vi "Add_sample_in_AO_DO_tasks_with_odd_number_of_samples.vi"(6 "Dummy Gate Waveform IN":waveform(i16), 7 "Black list (devices unable to output odd number of samples)":string[](array[string])=["PCI-6110"], 8 "error in (no error)":errorcluster, 9 "Gate Waveform (Digital) IN":digitalwaveform(waveform)={"t0"=timestamp(0 s since 1904-01-01), "dt"=0.0, "Y"={"transitions"=[], "data"=[]}, "error"={"status"=FALSE, "code"=37421928, "source"=""}}, 10 "Pockels Waveform IN":waveform(dbl), 11 "XY Waveform IN":waveform(dbl)[](array[waveform])) -> (0 "error out":errorcluster, 1 "Gate Waveform (Digital) OUT":digitalwaveform(waveform)={"t0"=timestamp(0 s since 1904-01-01), "dt"=0.0, "Y"={"transitions"=[], "data"=[]}, "error"={"status"=FALSE, "code"=37421928, "source"=""}}, 2 "Pockels Waveform OUT":waveform(dbl), 3 "XY Waveform OUT":waveform(dbl)[](array[waveform]), 4 "Dummy Gate Waveform OUT":waveform(i16), 5 "Sample added at the end of each task?":bool)   [LabVIEW 2012]
uses:
  GFG/GFGbooleanGet.vi
  GFG/GFGstringGet.vi
  <vilib>/Waveform/DWDTOps.llb/DWDT Digital Size.vi
  <vilib>/Waveform/WDTOps.llb/WDT Number of Waveform Samples DBL.vi
  <vilib>/Waveform/DWDTOps.llb/DWDT Digital to Boolean Array.vi
  <vilib>/Waveform/DTblOps.llb/DTbl Boolean Array to Digital.vi
  GFG/GFG library.lvlib
  <resource>/objmgr/daqmx.rc
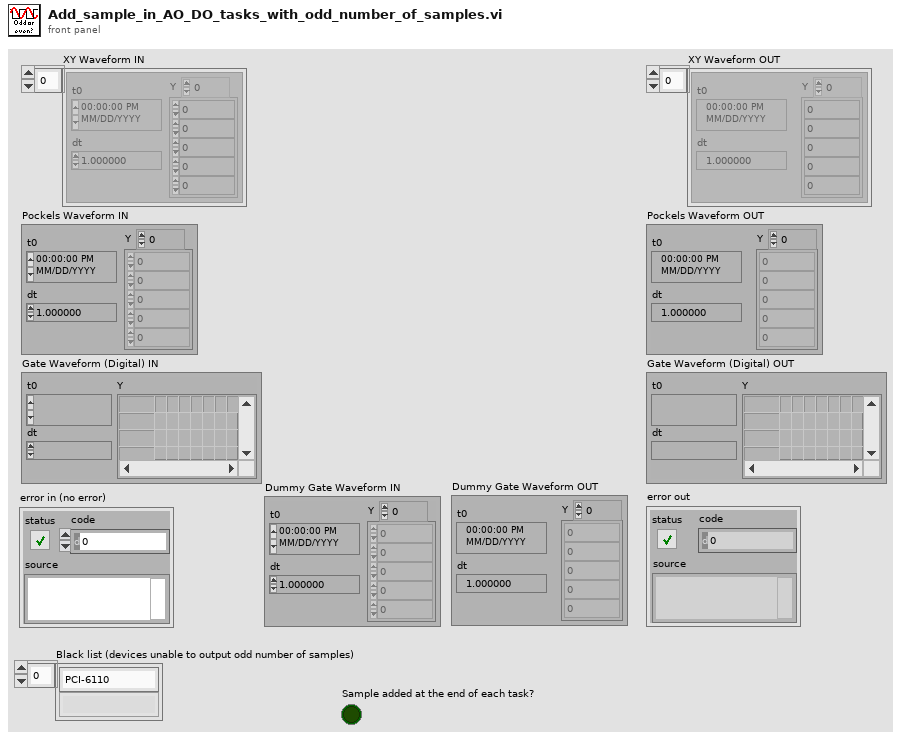
[diagram p1: front panel]
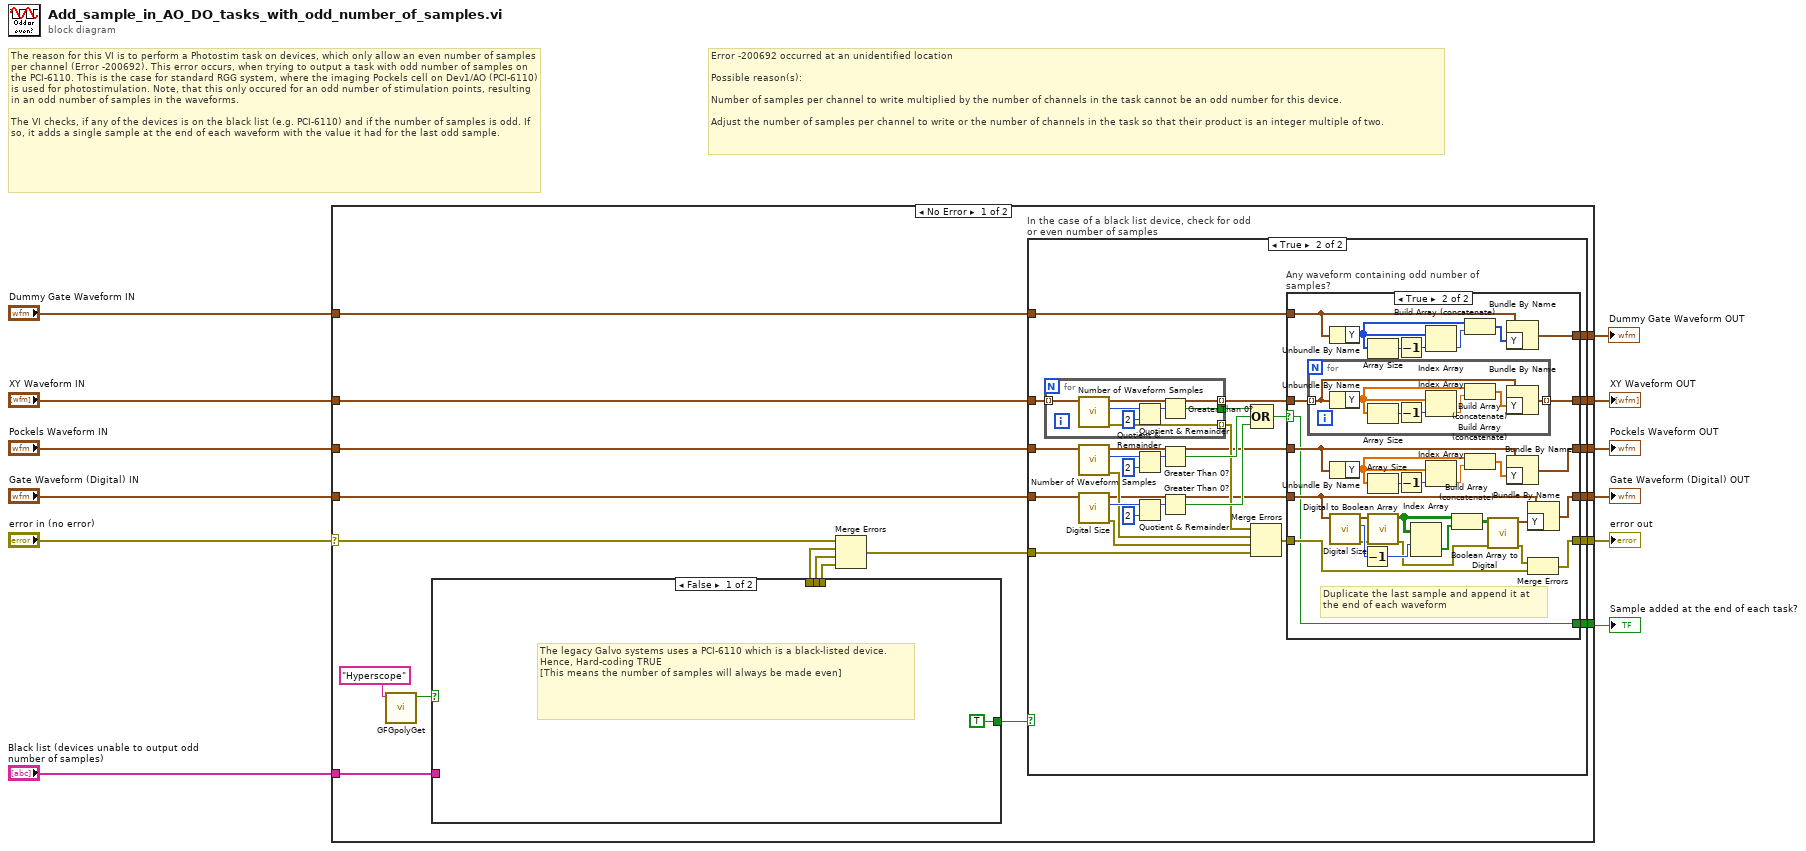
[diagram p0: block diagram]
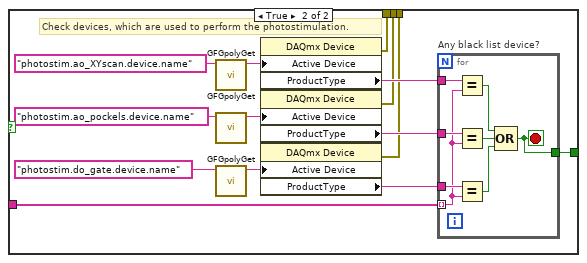
[diagram p2: hidden frame]
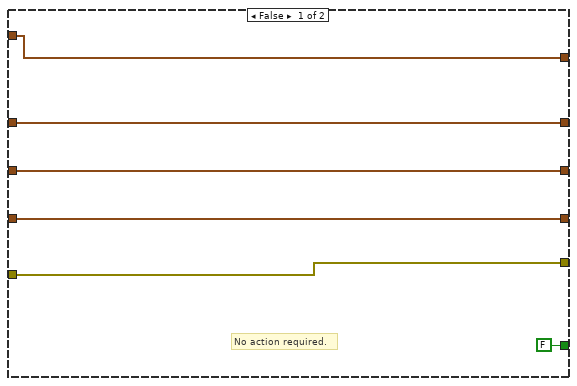
[diagram p3: hidden frame]
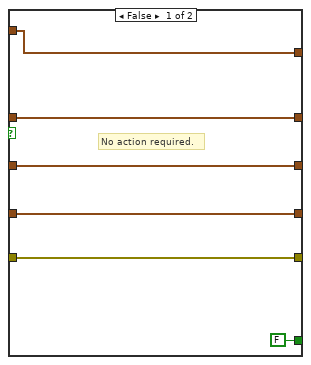
[diagram p4: hidden frame]
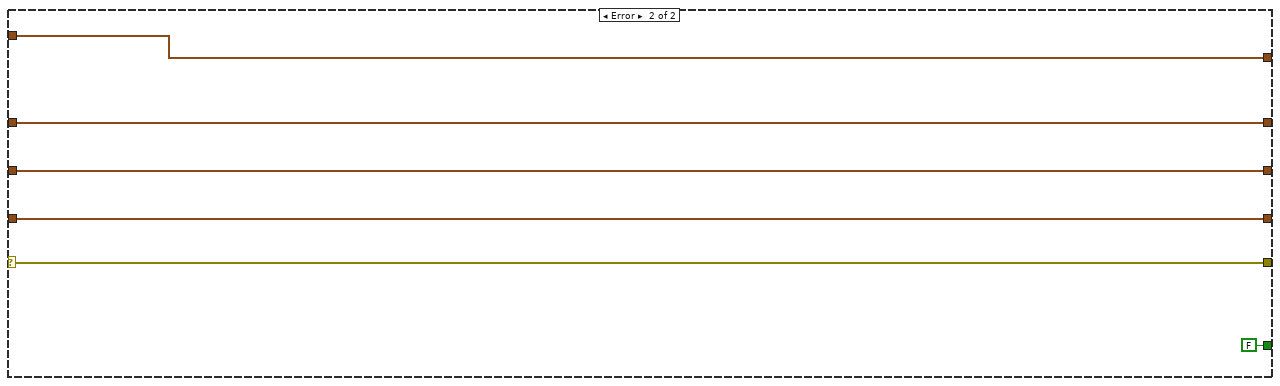
[diagram p5: hidden frame]
diagram:
  # "The reason for this VI is to perform a Photostim task on devices, which only allow an even number of samples per channel (Error -200692). This error occurs, when trying to output a task with odd number of samples on the PCI-6110. This is the case for standard RGG system, where the imaging Pockels cell on Dev1/AO (PCI-6110) is used for photostimulation. Note, that this only occured for an odd number of stimulation points, resulting in an odd number of samples in the waveforms.\n\nThe VI checks, if any of the devices is on the black list (e.g. PCI-6110) and if the number of samples is odd. If so, it adds a single sample at the end of each waveform with the value it had for the last odd sample."
  # "Error -200692 occurred at an unidentified location\n\nPossible reason(s):\n\nNumber of samples per channel to write multiplied by the number of channels in the task cannot be an odd number for this device. \n\nAdjust the number of samples per channel to write or the number of channels in the task so that their product is an integer multiple of two."
  n1 = case shown="No Error" "error in (no error)" {
    selector: "error in (no error)" -> [w27 w142]
    tunnel: "XY Waveform IN" -> [w26 w145]
    tunnel: "Pockels Waveform IN" -> [w25 w144]
    tunnel: "Gate Waveform (Digital) IN" -> [w24 w143]
    tunnel: [w22 w145] -> w11
    tunnel: [w21 w144] -> w10
    tunnel: [w20 w143] -> w9
    tunnel: [w19 w142] -> w8
    tunnel: "Black list (devices unable to output odd number of samples)" -> [w31 _]
    tunnel: [w17 FALSE] -> w3
    tunnel: "Dummy Gate Waveform IN" -> [w16 w140]
    tunnel: [w15 w140] -> w1
    frame No Error {
      n2 = call-poly "GFGpolyGet.vi"("Variable Name in"="Hyperscope") -> ("Boolean Value OUT"=w13:bool)  [unwired: 9 in, 1 out]
      n3 = case shown="False" w13 {
        tunnel: w31 -> [_ w40]
        tunnel: [_ w36] -> w30
        tunnel: [_ w35] -> w29
        tunnel: [_ w34] -> w28
        tunnel: [TRUE w33] -> w18
        frame False {
          # "The legacy Galvo systems uses a PCI-6110 which is a black-listed device. Hence, Hard-coding TRUE \n[This means the number of samples will always be made even]"
        }
        frame True {
          # "Check devices, which are used to perform the photostimulation."
          n4 = call-poly "GFGpolyGet.vi"("Variable Name in"="photostim.ao_XYscan.device.name") -> ("String"=w43:string)  [unwired: 9 in, 1 out]
          n5 = call-poly "GFGpolyGet.vi"("Variable Name in"="photostim.ao_pockels.device.name") -> ("String"=w42:string)  [unwired: 9 in, 1 out]
          n6 = call-poly "GFGpolyGet.vi"("Variable Name in"="photostim.do_gate.device.name") -> ("String"=w41:string)  [unwired: 9 in, 1 out]
          n7 = property class="DAQmx Device"("Active Device"=w43) -> (error out=w34:errorcluster, "ProductType"=w37:string)  [unwired: 2 in, 1 out]
          n8 = property class="DAQmx Device"("Active Device"=w42) -> (error out=w35:errorcluster, "ProductType"=w38:string)  [unwired: 2 in, 1 out]
          n9 = property class="DAQmx Device"("Active Device"=w41) -> (error out=w36:errorcluster, "ProductType"=w39:string)  [unwired: 2 in, 1 out]
          n10 = for "Any black list device?" {
            tunnel: w40 -> [w51] mode=indexing
            tunnel: w39 -> [w52]
            tunnel: w38 -> [w53]
            tunnel: w37 -> [w54]
            tunnel: [w47] -> w33
            stop <- w47 stop-if-true
            n11 = Equal?(x=w54, y=w51) -> (x = y?=w50:bool)
            n12 = Equal?(x=w53, y=w51) -> (x = y?=w49:bool)
            n13 = Equal?(x=w52, y=w51) -> (x = y?=w48:bool)
            n14 = Compound Arithmetic op=OR(w50, w49, w48) -> (w47:bool)
          }
        }
      }
      n15 = Merge Errors(w27, w28, w29, w30) -> (w23:errorcluster)
      n16 = case "In the case of a black list device, check for odd or even number of samples" shown="True" w18 {
        tunnel: w26 -> [w60 w88]
        tunnel: w25 -> [w59 w87]
        tunnel: w24 -> [w58 w86]
        tunnel: w23 -> [w57 w76]
        tunnel: [w60 w68] -> w22
        tunnel: [w59 w67] -> w21
        tunnel: [w58 w66] -> w20
        tunnel: [w57 w65] -> w19
        tunnel: [FALSE w63] -> w17
        tunnel: w16 -> [w55 w62]
        tunnel: [w55 w61] -> w15
        frame False {
          # "No action required."
        }
        frame True {
          n17 = for {
            tunnel: w88 -> [w139] mode=indexing
            tunnel: [w138] -> w71 mode=indexing
            tunnel: [w137] -> w72 mode=indexing
            tunnel: [w133] -> w64
            n18 = call-poly <vilib>:"Number of Waveform Samples.vi"("waveform in"=w139) -> ("error out"=w137:errorcluster, "number of samples"=w135:i32, "waveform out"=w138:waveform(dbl))  [unwired: 8 in]
            n19 = Quotient & Remainder(x=w135, y=2) -> (x-y*floor(x/y)=w134:i32)  [unwired: 1 out]
            n20 = Greater Than 0?(x=w134) -> (x > 0?=w133:bool)
          }
          n21 = call-poly <vilib>:"Number of Waveform Samples.vi"("waveform in"=w87) -> ("error out"=w74:errorcluster, "number of samples"=w84:i32, "waveform out"=w70:waveform(dbl))  [unwired: 8 in]
          n22 = call-poly <vilib>:"Digital Size.vi"("digital waveform in"=w86) -> ("error out"=w75:errorcluster, "number of samples"=w82:i32, "digital waveform out"=w69:digitalwaveform)  [unwired: 7 in, 1 out]
          n23 = Quotient & Remainder(x=w84, y=2) -> (x-y*floor(x/y)=w81:i32)  [unwired: 1 out]
          n24 = Quotient & Remainder(x=w82, y=2) -> (x-y*floor(x/y)=w80:i32)  [unwired: 1 out]
          n25 = Greater Than 0?(x=w81) -> (x > 0?=w79:bool)
          n26 = Greater Than 0?(x=w80) -> (x > 0?=w78:bool)
          n27 = Compound Arithmetic op=OR(w64, w79, w78) -> (w77:bool)
          n28 = Merge Errors(w72, w74, w75, w76) -> (w73:errorcluster)
          n29 = case "Any waveform containing odd number of samples?" shown="True" w77 {
            selector: w77 -> [_ w102]
            tunnel: w73 -> [w91 w105]
            tunnel: w71 -> [w94 w125]
            tunnel: w70 -> [w93 w108]
            tunnel: w69 -> [w92 w113]
            tunnel: [w94 w124] -> w68
            tunnel: [w93 w118] -> w67
            tunnel: [w92 w111] -> w66
            tunnel: [w91 w103] -> w65
            tunnel: [FALSE w102] -> w63
            tunnel: w62 -> [w89 w96]
            tunnel: [w89 w95] -> w61
            frame False {
              # "No action required."
            }
            frame True {
              # "Duplicate the last sample and append it at the end of each waveform"
              n30 = for {
                tunnel: w125 -> [w131] mode=indexing
                tunnel: [w127] -> w124 mode=indexing
                n31 = Unbundle By Name(w131) -> ("Y"=w129:dbl[])
                n32 = Array Size(array=w129) -> (size(s)=w132:i32)
                n33 = Decrement(x=w132) -> (x-1=w130:i32)
                n34 = Index Array(array=w129, index=w130) -> (element=w128:dbl)
                n35 = Build Array (concatenate)(w129, w128) -> (w126:dbl[])
                n36 = Bundle By Name(cluster=w131, "Y"=w126) -> (w127:waveform(dbl))
              }
              n37 = Unbundle By Name(w96) -> ("Y"=w99:i16[])
              n38 = Unbundle By Name(w108) -> ("Y"=w121:dbl[])
              n39 = call-poly <vilib>:"Digital Size.vi"("digital waveform in"=w113) -> ("error out"=w107:errorcluster, "number of samples"=w110:i32, "digital waveform out"=w114:digitalwaveform)  [unwired: 7 in, 1 out]
              n40 = Decrement(x=w110) -> (x-1=w109:i32)
              n41 = Array Size(array=w99) -> (size(s)=w101:i32)
              n42 = Array Size(array=w121) -> (size(s)=w119:i32)
              n43 = call-poly <vilib>:"Digital to Boolean Array.vi"("error in (no error)"=w107, "digital waveform"=w114) -> ("error out"=w106:errorcluster, "boolean array"=w117:bool[][])  [unwired: 8 in]
              n44 = Decrement(x=w101) -> (x-1=w100:i32)
              n45 = Decrement(x=w119) -> (x-1=w120:i32)
              n46 = Index Array(array=w117, index (row)=w109) -> (element=w116:bool[])  [unwired: 1 in]
              n47 = Index Array(array=w99, index=w100) -> (element=w98:i16)
              n48 = Index Array(array=w121, index=w120) -> (element=w122:dbl)
              n49 = Build Array (concatenate)(w117, w116) -> (w115:bool[][])
              n50 = Build Array (concatenate)(w99, w98) -> (w97:i16[])
              n51 = Build Array (concatenate)(w121, w122) -> (w123:dbl[])
              n52 = call-poly <vilib>:"Boolean Array to Digital.vi"("error in (no error)"=w106, "boolean array"=w115) -> ("error out"=w104:errorcluster, "digital data"=w112:digitaldata)  [unwired: 8 in]
              n53 = Bundle By Name(cluster=w96, "Y"=w97) -> (w95:waveform(i16))
              n54 = Bundle By Name(cluster=w108, "Y"=w123) -> (w118:waveform(dbl))
              n55 = Bundle By Name(cluster=w113, "Y"=w112) -> (w111:digitalwaveform)
              n56 = Merge Errors(w104, w105) -> (w103:errorcluster)
            }
          }
        }
      }
    }
    frame Error {
    }
  }
  "XY Waveform OUT" <- w11
  "Pockels Waveform OUT" <- w10
  "Gate Waveform (Digital) OUT" <- w9
  "Sample added at the end of each task?" <- w3
  "error out" <- w8
  "Dummy Gate Waveform OUT" <- w1
